vi "DataVis_ExtractScaleFromSortedSweepInfo.vi"(10 "Sorted Sweep Info in":T9 {"Sorted scan parameters"."?"."Rate" format="%.2f"; "Sorted scan parameters"."?"."Step" format="%#_6p"; "Sorted scan parameters"."?"."End" format="%#_6p"; "Sorted scan parameters"."?"."Start" format="%#_6p"}) -> (3 "X offset mult out":T1)   [LabVIEW 2016]
uses:
  <userlib>/LevyLab/Transport/SweepControl/Typedefs/ScanControl.ctl
  <userlib>/LevyLab/Transport/SweepControl/Typedefs/Cluster - ScanControl.ctl
  <userlib>/LevyLab/Transport/SweepControl/Typedefs/Enum - Priority.ctl
  <userlib>/LevyLab/Transport/SweepControl/Typedefs/Enum - Action.ctl
  <userlib>/LevyLab/Transport/SweepControl/Typedefs/ScanParamters.ctl
  <userlib>/LevyLab/Transport/SweepControl/Typedefs/Cluster - ScanParamters.ctl
  <userlib>/LevyLab/Transport/SweepControl/Typedefs/Enum - Experiments.ctl
  <vilib>/Utility/miscctls.llb/LVOffsetAndMultiplierTypeDef.ctl
  <userlib>/LevyLab/Transport/SweepControl/SweepControl.lvclass
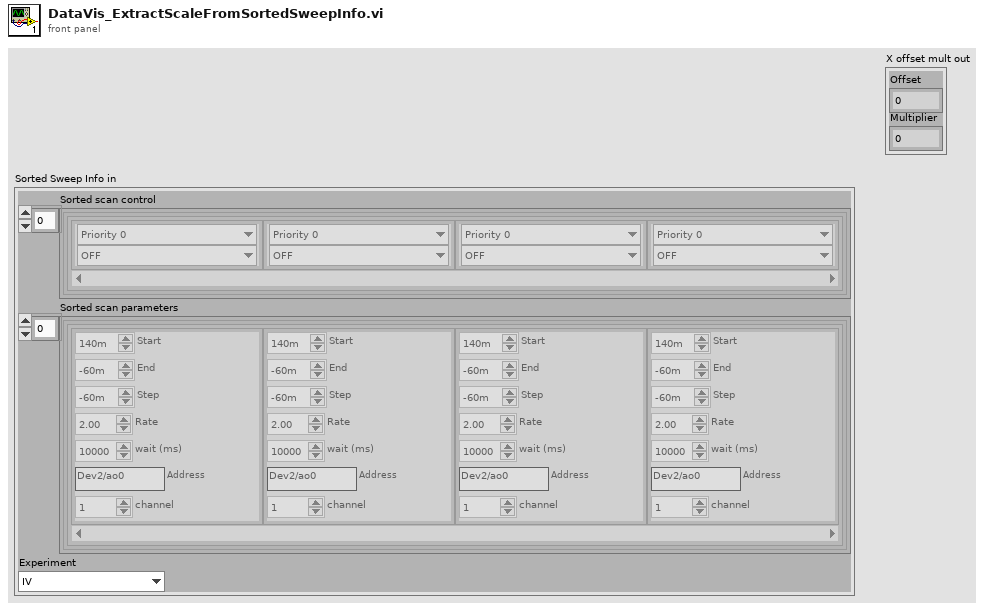
[diagram p1: front panel]
types:
  T1 = typedef "LVOffsetAndMultiplierTypeDef.ctl" = cluster{"Offset":dbl, "Multiplier":dbl}
  T2 = typedef "SweepControl.lvclass/ScanControl.ctl" = T3[]
  T3 = typedef "SweepControl.lvclass/Cluster - ScanControl.ctl" = cluster{"Priority":T4, "Scan name":T5}
  T4 = typedef "SweepControl.lvclass/Enum - Priority.ctl" = enum16{"Priority 0", "Priority 1", "Priority 2", "Priority 3", "Priority 4", "Priority 5"}
  T5 = typedef "SweepControl.lvclass/Enum - Action.ctl" = enum16{"OFF", "DSA_Vamp", "DSA_freq", "DSA_Vsg1", "DSA_Vsg2", "DSA_Vsg3", "DAQ_Vbg", "B_Field", "Humidity", "Temp", "MW_freq1", "MW_freq2", "MW_amplitude1", "MW_amplitude2"}
  T6 = typedef "SweepControl.lvclass/ScanParamters.ctl" = T7[]
  T7 = typedef "SweepControl.lvclass/Cluster - ScanParamters.ctl" = cluster{"Start":dbl, "End":dbl, "Step":dbl, "Rate":dbl, "wait (ms)":u32, "Address":string, "channel":i32}
  T8 = typedef "SweepControl.lvclass/Enum - Experiments.ctl" = enum16{"IV", "Lockin_time", "Lockin_Vsg", "Lockin (experimental)", "Lockin_Vsg_JKISM"}
  T9 = cluster{"Sorted scan control":cluster{T2}[], "Sorted scan parameters":cluster{T6}[], "Experiment":T8}
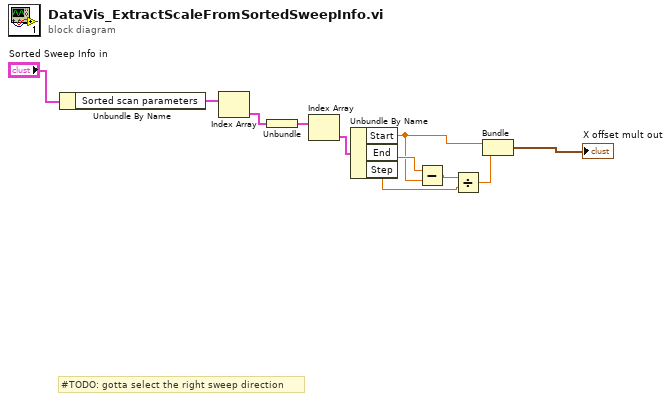
[diagram p0: block diagram]
diagram:
  # "#TODO: gotta select the right sweep direction"
  n1 = Unbundle By Name("Sorted Sweep Info in") -> ("Sorted scan parameters"=w10:cluster{T6}[])
  n2 = Index Array(array=w10) -> (element=w9:cluster{T6})  [unwired: 1 in]
  n3 = Unbundle(w9) -> (w8:T6)
  n4 = Index Array(array=w8) -> (element=w7:T7)  [unwired: 1 in]
  n5 = Unbundle By Name(w7) -> ("Start"=w5:dbl, "End"=w6:dbl, "Step"=w3:dbl)
  n6 = Subtract(x=w6, y=w5) -> (x-y=w4:dbl)
  n7 = Divide(x=w4, y=w3) -> (x/y=w2:dbl)
  n8 = Bundle("Start"=w5, w2) -> (→"X offset mult out":cluster{"Start":dbl, dbl})  [unwired: 1 in]
